vi "MatorInit.vi"(8 "错误输入（无错误）":errorcluster, 9 "Chan Ident":string="1", 10 "VISA资源名称":refnum<visa-resource-name>="COM1") -> (1 "InitStatus":bool)   [LabVIEW 2017]
panel:
  out "res_Homed":string
  out "res_Params":string
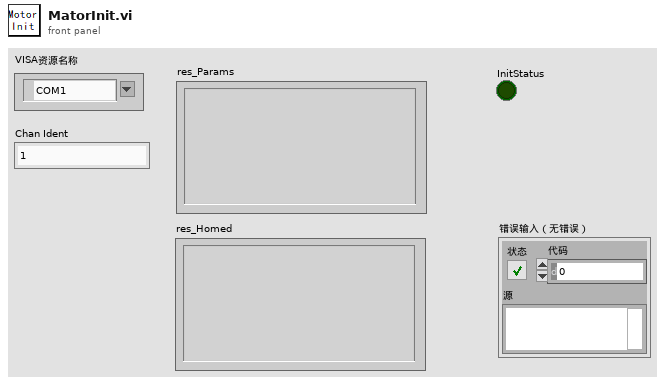
[diagram p1: front panel]
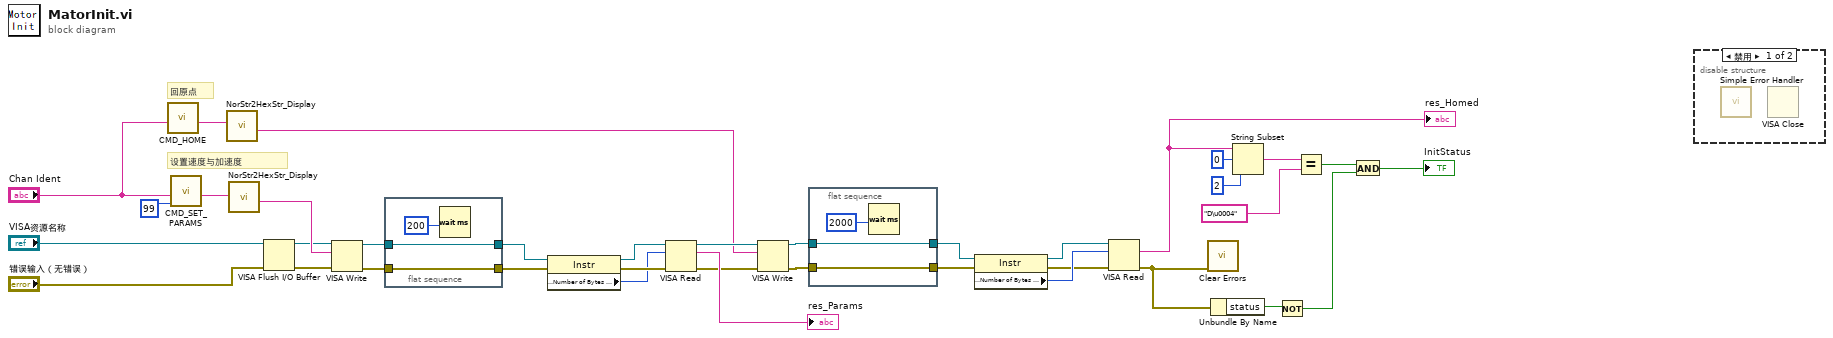
[diagram p0: block diagram]
diagram:
  # "设置速度与加速度"
  # "回原点"
  n1 = call "CMD_HOME.vi"("Chan Ident"="Chan Ident") -> ("Command"=w23:string)  [unwired: 10 in]
  n2 = call "CMD_SET_PARAMS.vi"("Max Vel"=99, "Chan Ident"="Chan Ident") -> ("ParamsCmd"=w27:string)  [unwired: 8 in, 1 out]
  n3 = call "NorStr2HexStr_Display.vi"("Normal Display"=w23) -> ("Hex Display"=w22:string)  [unwired: 10 in]
  n4 = call "NorStr2HexStr_Display.vi"("Normal Display"=w27) -> ("Hex Display"=w29:string)  [unwired: 10 in]
  n5 = VISA Flush I/O Buffer(VISA resource name="VISA资源名称", error in (no error)="错误输入（无错误）") -> (VISA resource name out=w5:refnum<visa-resource-name>, error out=w4:errorcluster)  [unwired: 1 in]
  n6 = VISA Write(VISA resource name=w5, write buffer=w29, error in (no error)=w4) -> (VISA resource name out=w35:refnum<visa-resource-name>, error out=w37:errorcluster)  [unwired: 1 out]
  n7 = flat-sequence {
    tunnel: w37 -> [w40]
    tunnel: [w40] -> w36
    tunnel: w35 -> [w39]
    tunnel: [w39] -> w34
    frame #0 {
      n8 = Wait (ms)(milliseconds to wait=u32 200 ("读取前延时(ms)")) -> ()  [unwired: 1 out]
    }
  }
  n9 = property class="Instr"(reference=w34, error in=w36) -> (reference out=w33:refnum<visa-resource-name>, error out=w32:errorcluster, "Serial Settings:Number of Bytes at Serial Port"=w30:u32)
  n10 = VISA Read(VISA resource name=w33, byte count=w30, error in (no error)=w32) -> (VISA resource name out=w26:refnum<visa-resource-name>, read buffer=→"res_Params":string, error out=w25:errorcluster)  [unwired: 1 out]
  n11 = VISA Write(VISA resource name=w26, write buffer=w22, error in (no error)=w25) -> (VISA resource name out=w16:refnum<visa-resource-name>, error out=w15:errorcluster)  [unwired: 1 out]
  n12 = flat-sequence {
    tunnel: w15 -> [w43]
    tunnel: [w43] -> w17
    tunnel: w16 -> [w42]
    tunnel: [w42] -> w18
    frame #0 {
      n13 = Wait (ms)(milliseconds to wait=u32 2000 ("读取前延时(ms)")) -> ()  [unwired: 1 out]
    }
  }
  n14 = property class="Instr"(reference=w18, error in=w17) -> (reference out=w19:refnum<visa-resource-name>, error out=w20:errorcluster, "Serial Settings:Number of Bytes at Serial Port"=w21:u32)
  n15 = VISA Read(VISA resource name=w19, byte count=w21, error in (no error)=w20) -> (read buffer=w10:string, error out=w3:errorcluster)  [unwired: 2 out]
  "res_Homed" <- w10
  n16 = call <vilib>:"Clear Errors.vi"("error in (no error)"=w3) -> ()  [unwired: 5 in, 2 out]
  n17 = Unbundle By Name(w3) -> ("status"=w9:bool)
  n18 = String Subset(string=w10, offset (0)=0 ("偏移量(0)"), length (rest)=2 ("长度（剩余）")) -> (substring=w12:string)
  n19 = Not(x=w9) -> (.not. x?=w7:bool)
  n20 = Equal?(x=w12, y="D\u0004") -> (x = y?=w8:bool)
  n21 = And(x=w8, y=w7) -> (x .and. y?=→"InitStatus":bool)
  n22 = disable-structure shown="禁用" {
    frame Disabled {
      n23 = call <vilib>:"Simple Error Handler.vi"() -> ()  [unwired: 2 in, 8 out]
      n24 = VISA Close() -> ()  [unwired: 2 in, 1 out]
    }
    frame Enabled {
    }
  }
